vi "Euler Function.vi"(6 "X":dbl[](array[numeric]) format="%.2f", 7 "time":dbl format="%.2f", 8 "result":dbl[][](array[numeric]) format="%.2f", 9 "table":i32[][][](array[numeric]), 10 "X":string[](array[string])=["x1", "x2"], 11 "time":string="t") -> (3 "F(X,time)":dbl[](array[numeric]) format="%.2f")   [LabVIEW 2020, in "NI_Gmath.lvlib"]
uses:
  <vilib>/gmath/NI_Gmath.lvlib
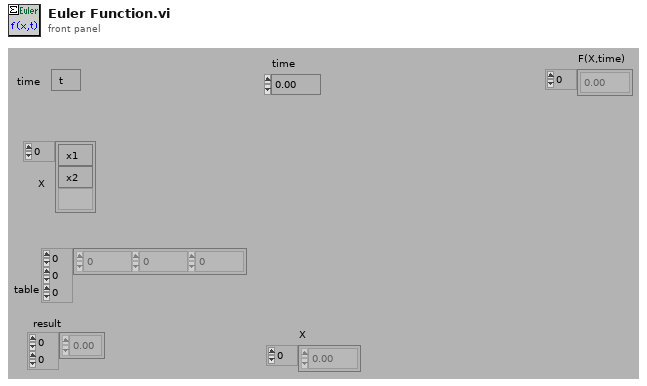
[diagram p1: front panel]
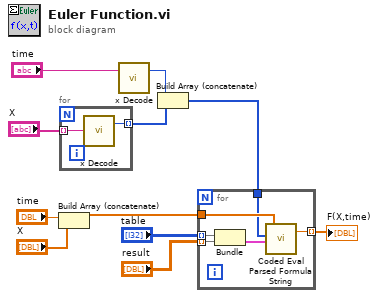
[diagram p0: block diagram]
diagram:
  n1 = Build Array (concatenate)("time", "X") -> (w10:dbl[])
  n2 = for {
    tunnel: "X" -> [w13] mode=indexing
    tunnel: [w12] -> w5 mode=indexing
    n3 = call <vilib>:"x Decode.vi"("x string"=w13) -> ("number"=w12:i32)  [unwired: 1 in, 1 out]
  }
  n4 = call <vilib>:"x Decode.vi"("x string"="time") -> ("number"=w9:i32)  [unwired: 1 in, 1 out]
  n5 = Build Array (concatenate)(w9, w5) -> (w8:i32[])
  n6 = for {
    tunnel: w8 -> [w17]
    tunnel: w10 -> [w18]
    tunnel: [w19] -> w7 mode=indexing
    tunnel: "result" -> [w15] mode=indexing
    tunnel: "table" -> [w14] mode=indexing
    n7 = Bundle("table"=w14, "result"=w15) -> (w16:cluster{"table":i32[][], "result":dbl[]})  [unwired: 1 in]
    n8 = call <vilib>:"Coded Eval Parsed Formula String.vi"("Parsed Formula"=w16, "Variables"=w17, "X Values"=w18) -> ("y value"=w19:dbl)  [unwired: 1 in, 1 out]
  }
  "F(X,time)" <- w7
